vi "Initialize.vi"(8 "error in (no error)":errorcluster, 10 "framework configuration":T1, 11 "Framework type":refnum<class "Framework.lvclass">) -> (0 "error out":errorcluster, 3 "Framework out":refnum<class "Framework.lvclass">)   [LabVIEW 2017, in "DSF Core.lvlib" / "Framework.lvclass"]
uses:
  Framework.lvclass
  DSF Configuration API/Public/Controls/DSF Engine Framework Configuration.ctl
  DSF Configuration API/Public/Controls/DSF Engine Plugin Configuration.ctl
  DSF Configuration API/Public/Controls/DSF Timing Info.ctl
  DSF Configuration API/Public/Controls/DSF Engine Transfer Group Configuration.ctl
  DSF Configuration API/Public/Controls/DSF Direction.ctl
  DSF Configuration API/Public/Controls/DSF Engine Transfer Configuration.ctl
  DSF Configuration API/Public/Controls/DSF Byte Order.ctl
  DSF Configuration API/Public/Controls/DSF Engine Channel Configuration.ctl
  DSF Configuration API/Public/Controls/DSF Data Type.ctl
  DSF Configuration API/Public/Controls/DSF Settings Info.ctl
  Thread/Thread Options.ctl
  Dispatcher/Dispatcher Thread.lvclass
  C:/Git/DSF/Data Sharing Framework/Source/Core/Engine/Classes/Thread/Thread.lvclass
  Thread/Plugin/Plugin Thread.lvclass
  Thread/Thread.lvclass
  DSF Core.lvlib
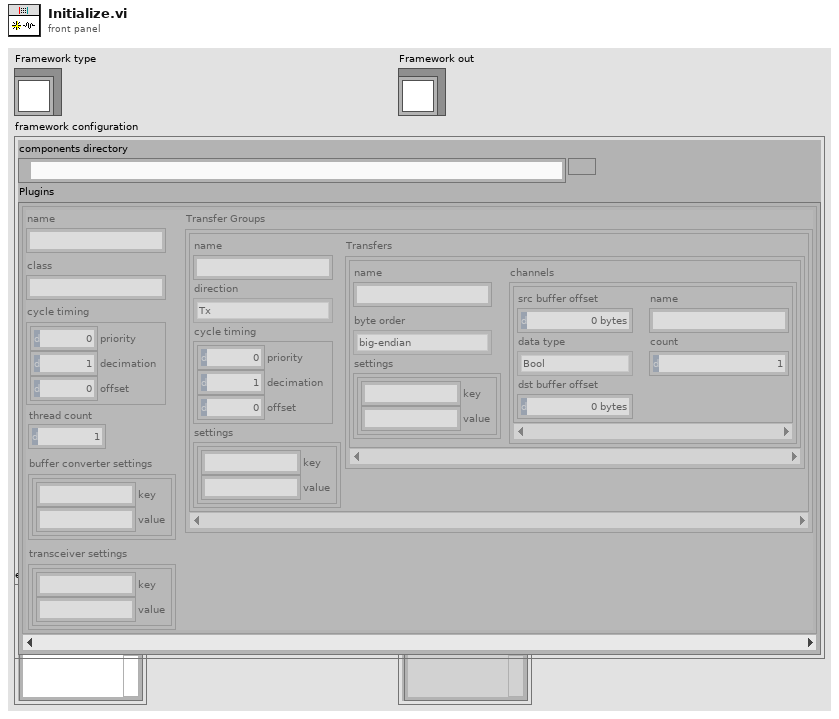
[diagram p1: front panel]
types:
  T1 = typedef "DSF Core.lvlib/DSF Engine Framework Configuration.ctl" = cluster{"components directory":path, "Plugins":T2[]}
  T2 = typedef "DSF Core.lvlib/DSF Engine Plugin Configuration.ctl" = cluster{"name":string, "class":string, "cycle timing":T3, "Transfer Groups":T4[], "thread count":i32, "buffer converter settings":T10, "transceiver settings":T10}
  T3 = typedef "DSF Core.lvlib/DSF Timing Info.ctl" = cluster{"priority":u64, "decimation":u64, "offset":u64}
  T4 = typedef "DSF Core.lvlib/DSF Engine Transfer Group Configuration.ctl" = cluster{"name":string, "direction":T5, "cycle timing":T3, "Transfers":T6[], "settings":T10}
  T5 = typedef "DSF Core.lvlib/DSF Direction.ctl" = enum8{"Tx", "Rx"}
  T6 = typedef "DSF Core.lvlib/DSF Engine Transfer Configuration.ctl" = cluster{"name":string, "byte order":T7, "channels":T8[], "settings":T10}
  T7 = typedef "DSF Core.lvlib/DSF Byte Order.ctl" = enum8{"big-endian", "little-endian"}
  T8 = typedef "DSF Core.lvlib/DSF Engine Channel Configuration.ctl" = cluster{"src buffer offset":u64, "name":string, "data type":T9, "count":u64, "dst buffer offset":u64}
  T9 = typedef "DSF Core.lvlib/DSF Data Type.ctl" = enum8{"Bool", "SGL", "DBL", "I8", "I16", "I32", "I64", "U8", "U16", "U32", "U64"}
  T10 = typedef "DSF Core.lvlib/DSF Settings Info.ctl" = cluster{"key":string, "value":string}[]
  T11 = typedef "DSF Core.lvlib/Thread.lvclass/Thread Options.ctl" = cluster{"Show FP On Call":bool, "Close FP After Call":bool}
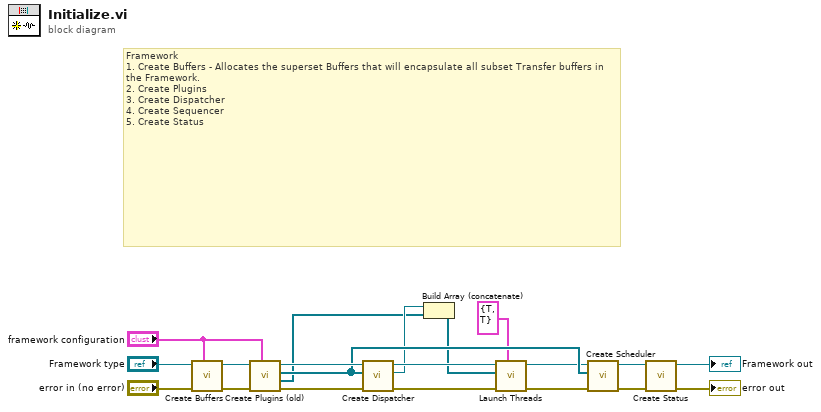
[diagram p0: block diagram]
diagram:
  # "Framework\n1. Create Buffers - Allocates the superset Buffers that will encapsulate all subset Transfer buffers in the Framework.\n2. Create Plugins\n3. Create Dispatcher\n4. Create Sequencer\n5. Create Status"
  n1 = call "Create Buffers.vi"("framework configuration"="framework configuration", "error in (no error)"="error in (no error)", "Framework in"="Framework type") -> ("error out"=w16:errorcluster, "Framework out"=w17:refnum<class "Framework.lvclass">)  [unwired: 7 in]
  n2 = call "Create Plugins (old).vi"("framework configuration"="framework configuration", "error in (no error)"=w16, "Framework in"=w17) -> ("error out"=w19:errorcluster, "Plugin Threads"=w1:refnum<class "Plugin Thread.lvclass">[], "Plugins"=w7:refnum<class "Plugin.lvclass">[], "Framework out"=w20:refnum<class "Framework.lvclass">)  [unwired: 5 in]
  n3 = call "Create Dispatcher.vi"("error in (no error)"=w19, "Plugins"=w7, "Framework in"=w20) -> ("error out"=w9:errorcluster, "Dispatcher Thread"=w2:refnum<class "Dispatcher Thread.lvclass">, "Framework out"=w6:refnum<class "Framework.lvclass">)  [unwired: 6 in]
  n4 = Build Array (concatenate)(w2, w1) -> (w3:refnum<class "Thread.lvclass">[])
  n5 = call "Launch Threads.vi"("options"=T11 {"Show FP On Call"=TRUE, "Close FP After Call"=TRUE}, "error in (no error)"=w9, "Threads"=w3, "Framework in"=w6) -> ("error out"=w8:errorcluster, "Framework out"=w5:refnum<class "Framework.lvclass">)  [unwired: 6 in]
  n6 = call "Create Scheduler.vi"("error in (no error)"=w8, "Plugins"=w7, "Framework in"=w5) -> ("error out"=w12:errorcluster, "Framework out"=w13:refnum<class "Framework.lvclass">)  [unwired: 7 in]
  n7 = call "Create Status.vi"("error in (no error)"=w12, "Framework in"=w13) -> ("error out"=→"error out":errorcluster, "Framework out"=→"Framework out":refnum<class "Framework.lvclass">)  [unwired: 8 in]
